vi "proiect.vi"(0 "ROI Descriptor (OCR/OCV 1)":T2={"Global Rectangle"=[427, 234, 1509, 910], "Contours"=[{"ID"=enum."External", "Type"=3, "Coordinates"=[427, 234, 1509, 910]}]} {"Contours"."Type" items=["No Selection", "Point", "Line", "Rectangle", "Oval", "Polygon", "Freehand Region", "Annulus", "Unused2", "Unused3", "Broken Line", "Freehand Line", "Rotated Rectangle"]}, 1 "File Path (OCR/OCV 1)":path=path "D:/snd/proiect/setcaractere.abc", 2 "Parameters (OCR/OCV 1)":T1={"Threshold Data"={"Method"=enum."Uniform", "Looking for"=1, "Color Mode"=0, "Kernel Size"={"Width"=32, "Height"=32}, "Ranges"=[{"Min"=1, "Max"=255}]}, "Reject Border"=TRUE, "Number Of Erosions"=0, "Size & Spacing"={"Segment Algorithm"=0, "Min Bounding Rect Width"=1, "Max Bounding Rect Width"=65536, "Min Bounding Rect Height"=1, "Max Bounding Rect Height"=65536, "Min Character Size"=20, "Max Character Size"=65536, "Min Char Spacing"=1, "Max Horiz Element Spacing"=1, "Max Vert Element Spacing"=0, "Max Space Distance"=65536}, "Read Options"={"Read Strategy"=1, "Read Resolution"=2, "Scale Dependant"=FALSE, "Aspect Ratio"=400, "Acceptance Level"=700, "Substitution Character"="?", "MultiLine"=TRUE}, "Valid Characters"=[], "Use Text Pattern"=FALSE, "Orientation"=0, "# Lines Expected"=10, "Number of Blocks"=4} {"Threshold Data"."Looking for" items=["Light on Dark", "Dark on Light"]; "Threshold Data"."Color Mode" items=["RGB", "HSL", "HSV", "HSI"]; "Size & Spacing"."Segment Algorithm" items=["None", "Shortest Segment", "Legacy Auto Split"]; "Read Options"."Read Strategy" items=["Aggressive", "Conservative"]; "Read Options"."Read Resolution" items=["Low", "Medium", "High"]; "Valid Characters"."Pre-defined characters" items=["Any Character", "User-defined Characters", "Alphabetic", "Alphanumeric", "Uppercase Letters", "Lowercase Letters", "Decimal Digits", "Hexadecimal Digits", "Pattern", "Force Space"]; "Orientation" items=["Baseline inside", "Baseline outside"]}, 7 "error in":errorcluster) -> (20 "String (OCR/OCV 1)":string, 21 "OCR Session (OCR/OCV 1)":T4, 27 "error out":errorcluster)   [LabVIEW 2018]
uses:
  <vilib>/vision/OCR.llb/IMAQ OCR Session.ctl
  <vilib>/addons/database/Connection.llb/DB Tools Open Connec (Path).vi
  <vilib>/vision/NI_Vision_Development_Module.lvlib
  <vilib>/addons/database/NI_Database_API.lvlib
panel:
  in  "Citeste":bool
  in  "connection information":path
  out "Image Out":T3(plugin-control)
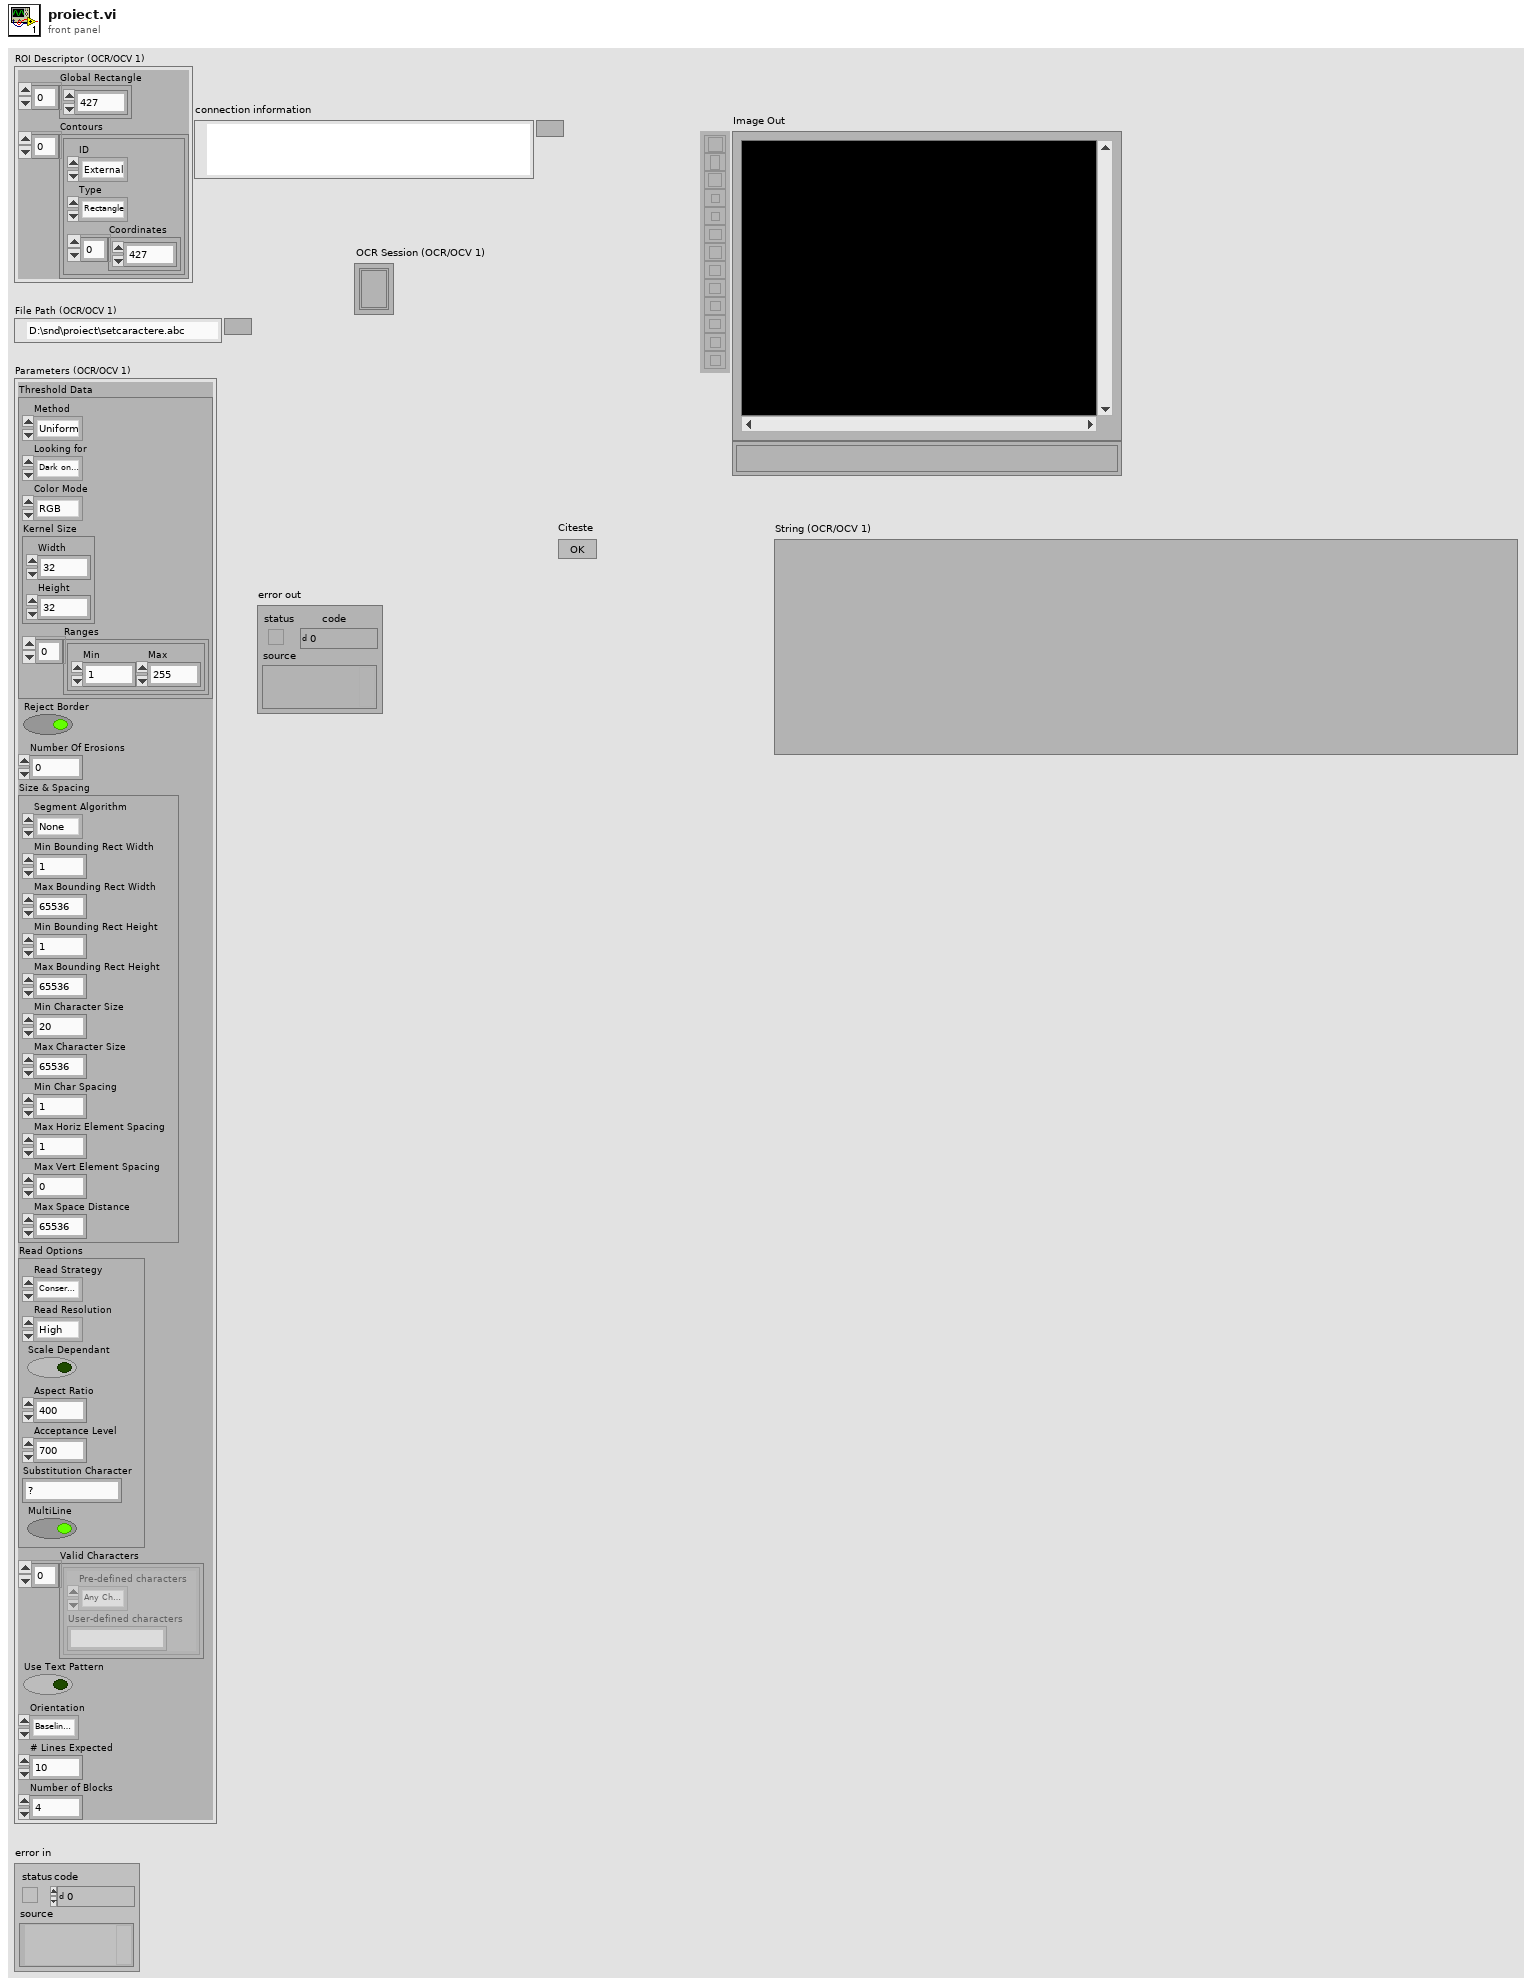
[diagram p1: front panel]
types:
  T1 = cluster{"Threshold Data":cluster{"Method":enum16{"Fixed Range", "Uniform", "Linear", "Non Linear", "Local", "Color"}, "Looking for":u32, "Color Mode":u32, "Kernel Size":cluster{"Width":i32, "Height":i32}, "Ranges":cluster{"Min":i32, "Max":i32}[]}, "Reject Border":bool, "Number Of Erosions":i32, "Size & Spacing":cluster{"Segment Algorithm":u16, "Min Bounding Rect Width":i32, "Max Bounding Rect Width":i32, "Min Bounding Rect Height":i32, "Max Bounding Rect Height":i32, "Min Character Size":i32, "Max Character Size":i32, "Min Char Spacing":i32, "Max Horiz Element Spacing":i32, "Max Vert Element Spacing":i32, "Max Space Distance":i32}, "Read Options":cluster{"Read Strategy":i32, "Read Resolution":i32, "Scale Dependant":bool, "Aspect Ratio":i32, "Acceptance Level":i32, "Substitution Character":string, "MultiLine":bool}, "Valid Characters":cluster{"Pre-defined characters":i32, "User-defined characters":string}[], "Use Text Pattern":bool, "Orientation":u32, "# Lines Expected":u32, "Number of Blocks":i32}
  T2 = cluster{"Global Rectangle":i32[], "Contours":cluster{"ID":enum32{"External", "Internal"}, "Type":u32, "Coordinates":i32[]}[]}
  T3 = typedef "IMAQ Image.ctl" = refnum<image>
  T4 = typedef "IMAQ OCR Session.ctl" = refnum<k1>
  T5 = typedef "Image Type" = u32
  T6 = typedef "NI_Database_API.lvlib/Conn ObjectReference.ctl" = refnum<k1>
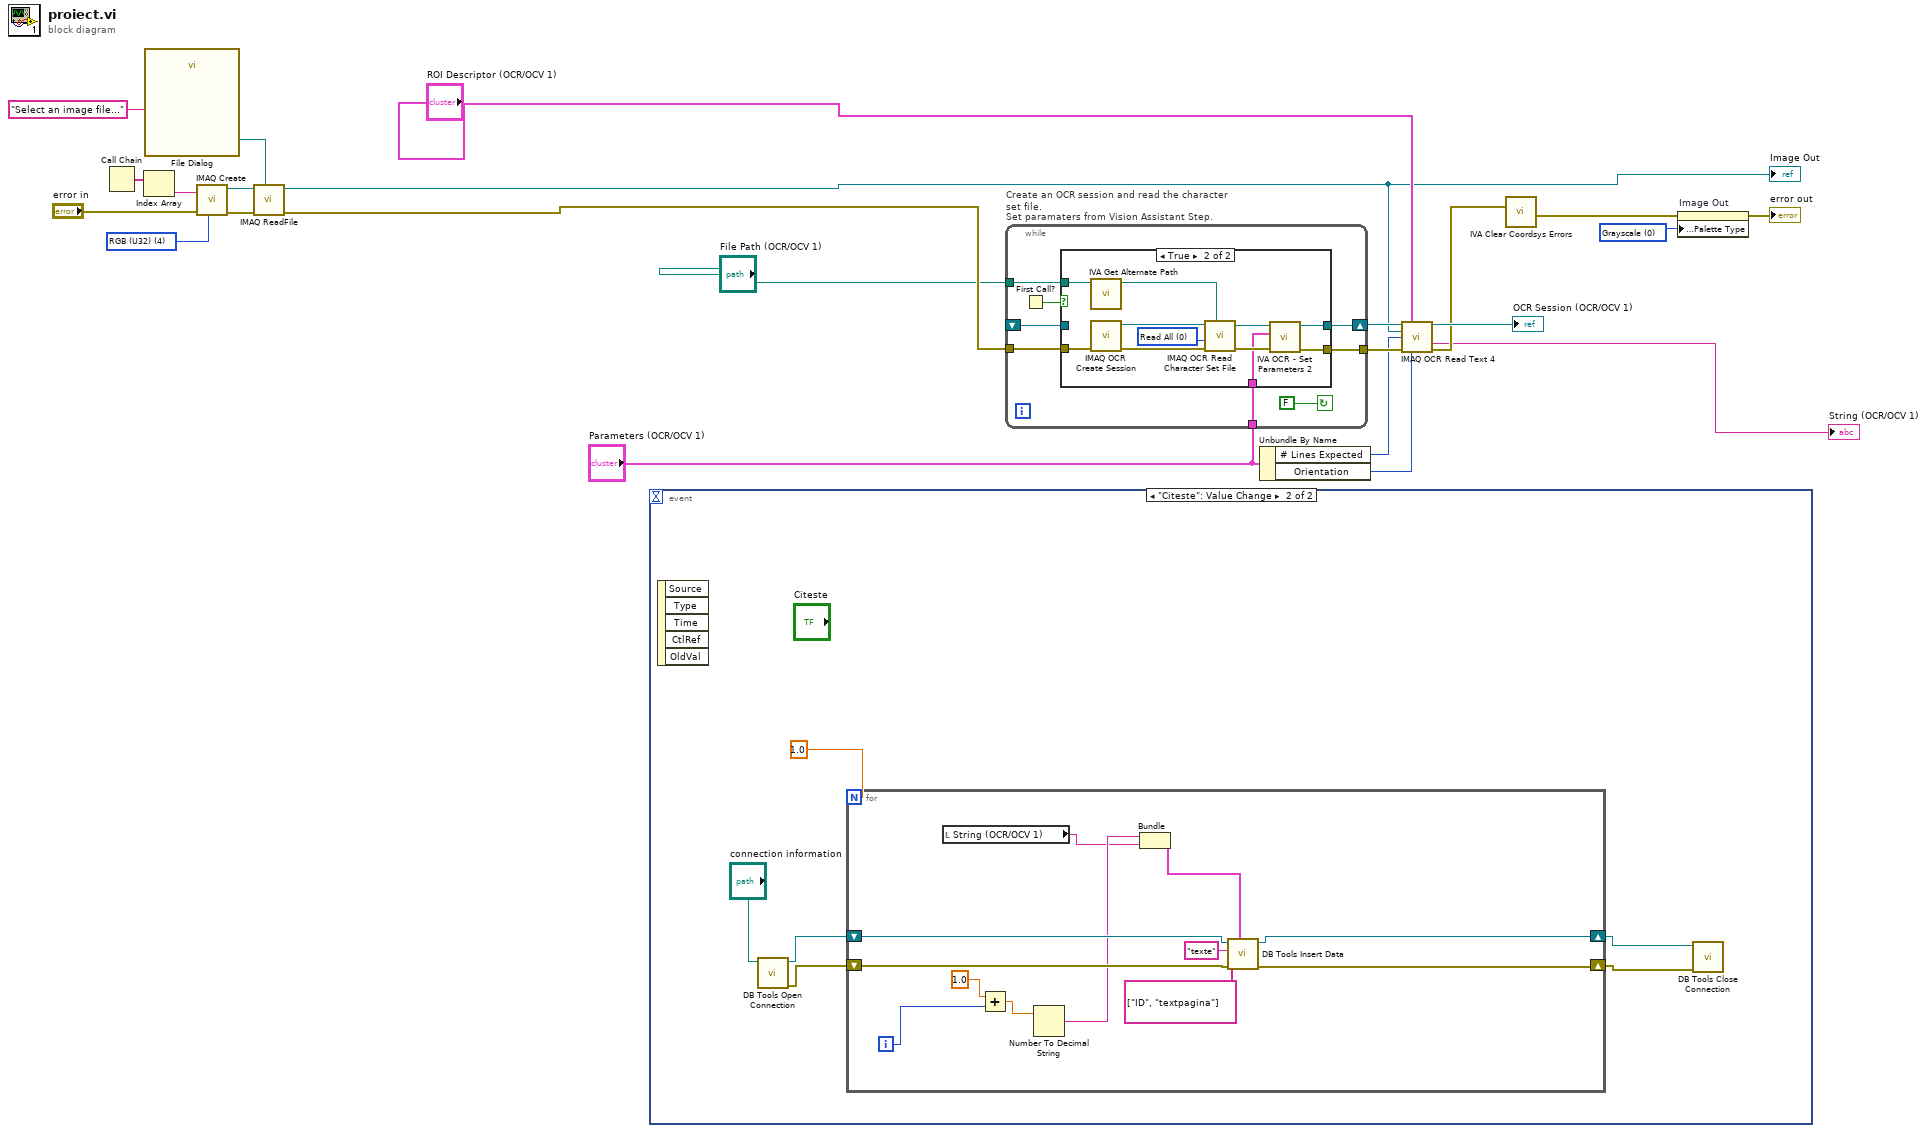
[diagram p0: block diagram]
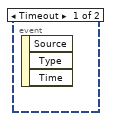
[diagram p2: hidden frame]
diagram:
  w2 = u32 0 items=["Grayscale", "Binary", "Gradient", "Rainbow", "Temperature", "User Defined", "Binary 16 Bit", "Gradient 16 Bit", "Rainbow 16 Bit", "Temperature 16 Bit", "User Defined 16 Bit"] ("Palette Type")
  w15 = T5 4 items=["Grayscale (U8)", "Grayscale (I16)", "Grayscale (SGL)", "Complex (CSG)", "RGB (U32)", "HSL (U32)", "RGB (U64)", "Grayscale (U16)"] ("Image Type")
  n1 = Call Chain() -> (call chain=w19:string[])
  n2 = Index Array(array=w19) -> (element=w18:string)  [unwired: 1 in]
  n3 = call "File Dialog"("prompt"="Select an image file...") -> ("selected path"=w16:path)  [unwired: 6 in, 8 out]
  n4 = call "IMAQ Create"("Image Name"=w18, "Image Type"=w15, "error in (no error)"="error in") -> ("New Image"=w22:T3, "error out"=w21:errorcluster)  [unwired: 1 in, 1 out]
  n5 = call "IMAQ ReadFile"("File Path"=w16, "error in (no error)"=w21, "Image"=w22) -> ("error out"=w23:errorcluster, "Image Out"=w3:T3)  [unwired: 2 in, 5 out]
  "Image Out" <- w3
  n6 = event shown="[1] \"Citeste\": Value Change" {
    selector: _ -> [_ _]
    dyn-events: _ -> [_ _]
    timeout: _ -> [_ _]
    event Timeout {
      n7 = event-data() -> ()  [unwired: 1 in, 3 out]
    }
    event "Citeste": Value Change {
      n8 = event-data() -> ()  [unwired: 1 in, 5 out]
      n9 = call-poly <vilib>:"DB Tools Open Connection.vi"("connection information"="connection information") -> ("error out"=w27:errorcluster, "connection reference"=w26:T6)  [unwired: 7 in]
      n10 = for {
        N: 1.0 -> [_]
        shift-right: [w36] -> w25
        shift-left: w26 -> [w37]
        shift-right: [w35] -> w24
        shift-left: w27 -> [w38]
        i -> [w41]
        n11 = local read "String (OCR/OCV 1)"() -> (w30:string)
        n12 = Add(x=1.0, y=w41) -> (x+y=w32:dbl)
        n13 = Number To Decimal String(number=w32) -> (decimal integer string=w31:string)  [unwired: 1 in]
        n14 = Bundle(w31, "String (OCR/OCV 1)"=w30) -> (w39:cluster{string, "String (OCR/OCV 1)":string})  [unwired: 1 in]
        n15 = call <vilib>:"DB Tools Insert Data.vi"("data"=w39, "error in (no error)"=w38, "columns"=string[] ["ID", "textpagina"], "table"="texte", "connection reference"=w37) -> ("error out"=w35:errorcluster, "connection reference out"=w36:T6)  [unwired: 5 in]
      }
      n16 = call <vilib>:"DB Tools Close Connection.vi"("error in (no error)"=w24, "connection reference"=w25) -> ()  [unwired: 5 in, 1 out]
    }
  }
  n17 = while "Create an OCR session and read the character set file.\nSet paramaters from Vision Assistant Step." {
    shift-right: [w46] -> w9
    shift-left: _ -> [w45]
    tunnel: w23 -> [w48]
    tunnel: "Parameters (OCR/OCV 1)" -> [w44]
    tunnel: "File Path (OCR/OCV 1)" -> [w43]
    tunnel: [w42] -> w10
    stop <- FALSE continue-if-true
    n18 = First Call?() -> (First Call?: T/F=w47:bool)
    n19 = case shown="True" w47 {
      tunnel: w43 -> [_ w55]
      tunnel: w48 -> [w50 w59]
      tunnel: [w51 w57] -> w46
      tunnel: [w50 w56] -> w42
      tunnel: w44 -> [_ w52]
      tunnel: w45 -> [w51 _]
      frame False {
      }
      frame True {
        w60 = 0 items=["Read All", "Read Character Set Only", "Read Properties Only"] ("Read Options")
        n20 = call <vilib>:"IVA Get Alternate Path.vi"("Path In"=w55) -> ("Path Out"=w54:path)  [unwired: 10 out]
        n21 = call "IMAQ OCR Create Session"("error in (no error)"=w59) -> ("error out"=w61:errorcluster, "IMAQ OCR Session"=w62:T4)  [unwired: 9 out]
        n22 = call "IMAQ OCR Read Character Set File"("File Path"=w54, "error in (no error)"=w61, "Read Options"=w60, "IMAQ OCR Session"=w62) -> ("error out"=w58:errorcluster, "IMAQ OCR Session (dup)"=w53:T4)  [unwired: 1 in, 5 out]
        n23 = call <vilib>:"IVA OCR - Set Parameters 2.vi"("error in (no error)"=w58, "Parameters"=w52, "IMAQ OCR Session"=w53) -> ("error out"=w56:errorcluster, "IMAQ OCR Session Out"=w57:T4)  [unwired: 7 in]
      }
    }
  }
  n24 = Unbundle By Name("Parameters (OCR/OCV 1)") -> ("# Lines Expected"=w7:u32, "Orientation"=w8:u32)
  n25 = call "IMAQ OCR Read Text 4"("IMAQ OCR Session"=w9, "ROI Descriptor"="ROI Descriptor (OCR/OCV 1)", "Image"=w3, "Number of Lines Requested"=w7, "error in (no error)"=w10, "Orientation"=w8) -> ("IMAQ OCR Session (dup)"=→"OCR Session (OCR/OCV 1)":T4, "Read String"=→"String (OCR/OCV 1)":string, "error out"=w6:errorcluster)  [unwired: 7 out]
  n26 = call <vilib>:"IVA Clear Coordsys Errors.vi"("error in (no error)"=w6) -> ("error out"=w5:errorcluster)  [unwired: 10 in]
  n27 = property on="Image Out" class="ImageControl"(error in=w5, "Palette:Palette Type"=w2) -> (error out=→"error out":errorcluster)  [unwired: 1 in, 1 out]
